vi "readConfigEvt.vi"(8 "error in (no error)":errorcluster, 11 "Path in":T1) -> (0 "error out":errorcluster, 2 "regEvt":string[][](array[string]), 3 "Path out":T1)   [LabVIEW 2018]
doc: "Read events from default.ini file that will be registered by TCP Server.\n\nNOTE: this is only for internal use. User does not call this function directly."
uses:
  <vilib>/Utility/config.llb/Config Data RefNum.ctl
  <vilib>/Utility/config.llb/NI_LVConfig.lvlib
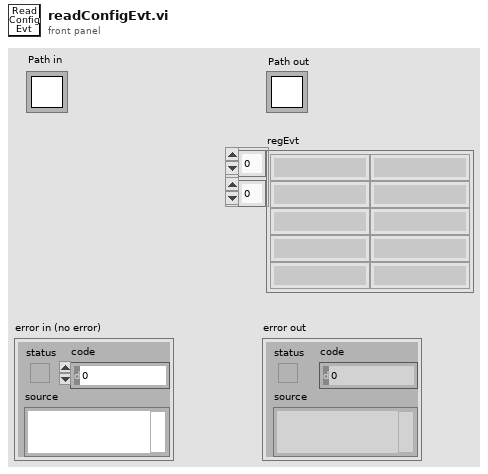
[diagram p1: front panel]
types:
  T1 = typedef "NI_LVConfig.lvlib/Config Data RefNum.ctl" = refnum<k1>
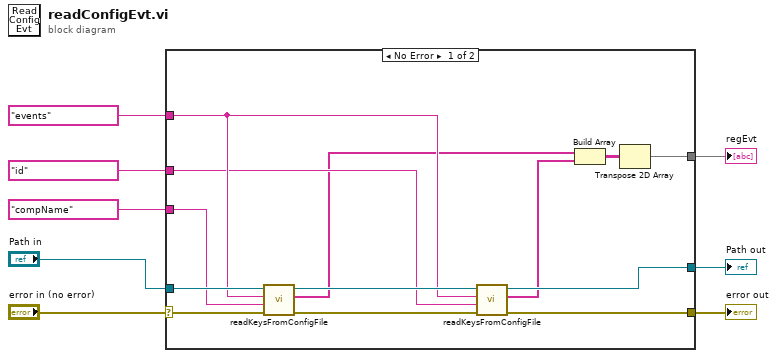
[diagram p0: block diagram]
diagram:
  n1 = case shown="No Error" "error in (no error)" {
    selector: "error in (no error)" -> [w21 w23]
    tunnel: "compName" -> [w14 _]
    tunnel: "events" -> [w16 _]
    tunnel: [w18 w23] -> w6
    tunnel: "Path in" -> [w20 w22]
    tunnel: [w15 w22] -> w4
    tunnel: [w13 _] -> w2
    tunnel: "id" -> [w12 _]
    frame No Error {
      n2 = call "readKeysFromConfigFile.vi"("error in (no error)"=w21, "keys"=w14, "section"=w16, "Refnum in"=w20) -> ("error out"=w19:errorcluster, "arrayOfKeys"=w11:string[], "Refnum out"=w17:T1)  [unwired: 5 in]
      n3 = call "readKeysFromConfigFile.vi"("error in (no error)"=w19, "keys"=w12, "section"=w16, "Refnum in"=w17) -> ("error out"=w18:errorcluster, "arrayOfKeys"=w10:string[], "Refnum out"=w15:T1)  [unwired: 5 in]
      n4 = Build Array(w11, w10) -> (w9:string[][])
      n5 = Transpose 2D Array(2D array=w9) -> (transposed array=w13:string[][])
    }
    frame Error {
    }
  }
  "regEvt" <- w2
  "error out" <- w6
  "Path out" <- w4
